vi "CheckIfSetCommand.vi"(0 "Command":string) -> (1 "setCommand?":bool, 2 "getCommand?":bool, 3 "variable":string)   [LabVIEW 2011]
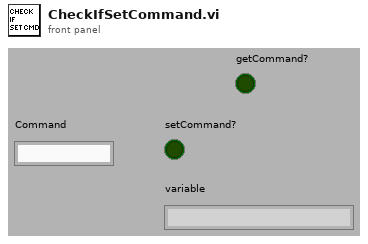
[diagram p1: front panel]
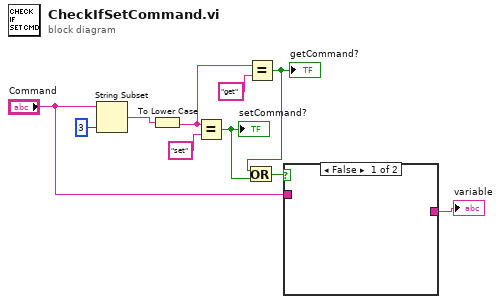
[diagram p0: block diagram]
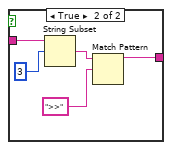
[diagram p2: hidden frame]
diagram:
  n1 = String Subset(string="Command", length (rest)=3 ("length (rest)")) -> (substring=w9:string)  [unwired: 1 in]
  n2 = To Lower Case(string=w9) -> (all lower case string=w7:string)
  n3 = Equal?(x=w7, y="set") -> (x = y?=w3:bool)
  "setCommand?" <- w3
  n4 = Equal?(x=w7, y="get") -> (x = y?=w2:bool)
  "getCommand?" <- w2
  n5 = Or(x=w2, y=w3) -> (x .or. y?=w1:bool)
  n6 = case shown="False" w1 {
    tunnel: "Command" -> [_ w15]
    tunnel: [_ w12] -> w4
    frame False {
    }
    frame True {
      n7 = String Subset(string=w15, offset (0)=3 ("length (rest)")) -> (substring=w14:string)  [unwired: 1 in]
      n8 = Match Pattern(string=w14, regular expression=">>") -> (before substring=w12:string)  [unwired: 1 in, 3 out]
    }
  }
  "variable" <- w4
